vi "build.maps.vi"(8 "error in (no error)":errorcluster, 10 "manager_daemon.lvclass":refnum<class "manager_daemon.lvclass">, 11 "paths":T1={"issue map path"=path "D:/Comics/data/key_maps/issues.bin", "char map path"=path "D:/Comics/data/key_maps/chars.bin", "concept map path"=path "D:/Comics/data/key_maps/concepts.bin", "story map path"=path "D:/Comics/data/key_maps/storys.bin", "team map path"=path "D:/Comics/data/key_maps/teams.bin", "volume map path"=path "D:/Comics/data/key_maps/volumes.bin", "volumes path"=path "D:/Comics/data/cv_volumes", "issues path"=path "D:/Comics/data/cv_issues", "folder map path"=path ""}) -> (0 "error out":errorcluster)   [LabVIEW 2024, in "manager_daemon.lvclass"]
uses:
  manager_daemon/manager_daemon.lvclass
  manager_daemon/type_defs/paths--cluster.ctl
  manager_daemon/type_defs/IssueData--clustrer.ctl
  manager_daemon/type_defs/VolumeData--cluster.ctl
  CV_Shared_Library/volume.type--enum.ctl
  manager_daemon/type_defs/sub-map--map.ctl
  manager_daemon/type_defs/SubData--cluster.ctl
  manager_daemon/private/add.sub.to.map.vi
  CV_Shared_Library/open.local.issue.file.vi
  CV_Shared_Library/open.local.volume.file.vi
  CV_Shared_Library/CV_Shared_Library.lvlib
panel:
  out "total volumes":i32
  out "volume progress":i32(slide) scale=0.0..5644.0
  out "total issues":i32
  out "issue progress":i32(slide) scale=0.0..45513.0
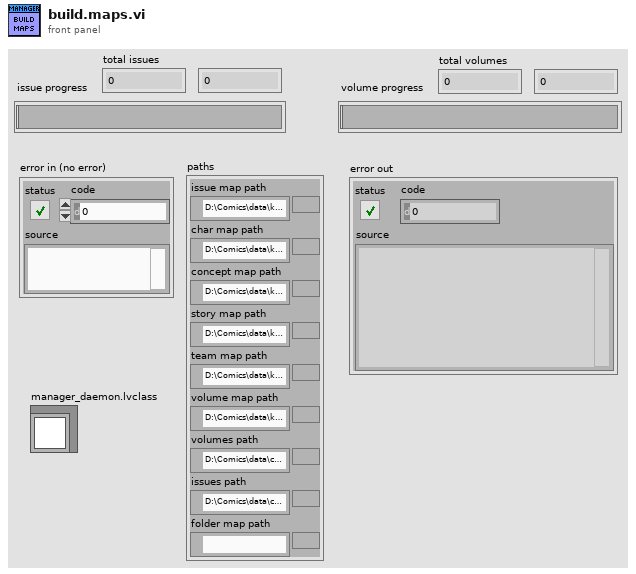
[diagram p1: front panel]
types:
  T1 = typedef "manager_daemon.lvclass/paths--cluster.ctl" = cluster{"issue map path":path, "char map path":path, "concept map path":path, "story map path":path, "team map path":path, "volume map path":path, "volumes path":path, "issues path":path, "folder map path":path}
  T2 = typedef "manager_daemon.lvclass/sub-map--map.ctl" = map{string, T3}
  T3 = typedef "manager_daemon.lvclass/SubData--cluster.ctl" = cluster{"id":i32, "issues":set{i32}}
  T4 = typedef "manager_daemon.lvclass/VolumeData--cluster.ctl" = cluster{"name":string, "sortable_name":string, "aliases":string[], "description":string, "site_detail_url":string, "count_of_issues":i32, "start_year":i32, "publisher_id":i32, "issue_ids":i32[], "date_last_updated":timestamp, "volume":i32, "cv_id":string, "volume type":T5, "source_path":path}
  T5 = typedef "CV_Shared_Library.lvlib/volume.type--enum.ctl" = enum16{"Ongoing", "Limited Series", "Annual", "One Shot", "Reprint/Document", "Star Comics", "Epic Comics"}
  T6 = typedef "manager_daemon.lvclass/IssueData--clustrer.ctl" = cluster{"cover_date":timestamp, "cv_id":string, "name":string, "sortable_name":string, "issue_number":string, "deck":string, "description":string, "id":i32, "store_date":timestamp, "date_last_updated":timestamp, "site_detail_url":string, "cover_url":string, "source_path":path}
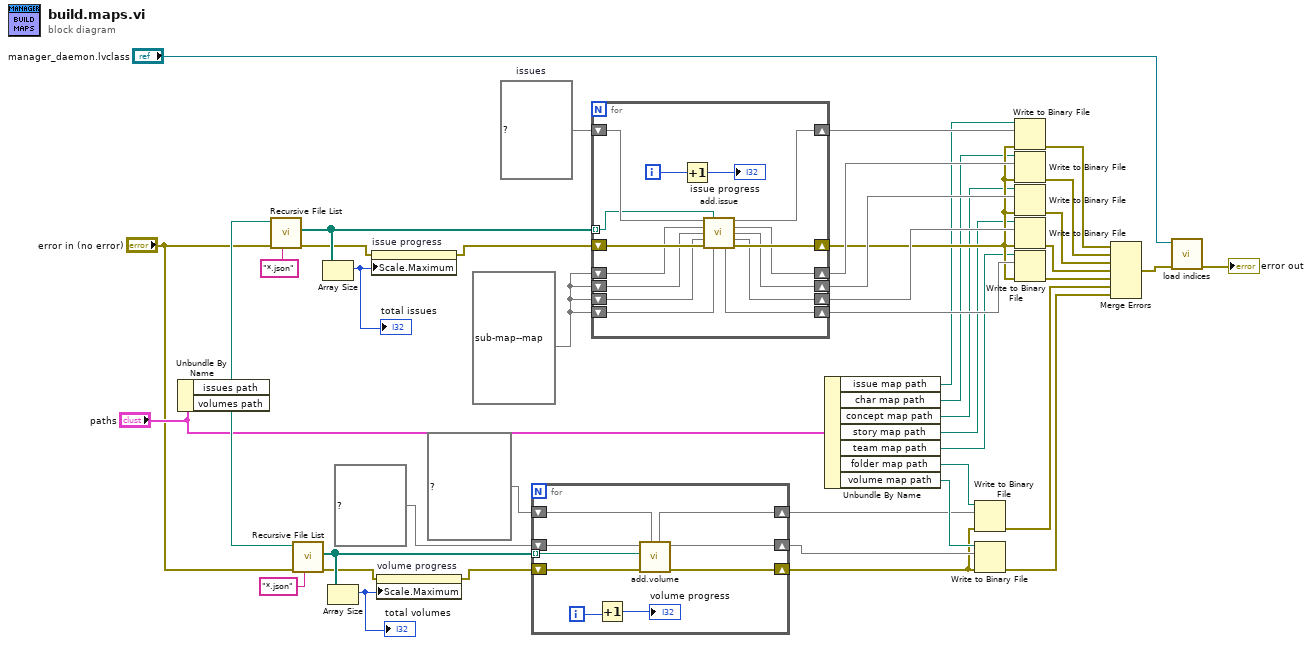
[diagram p0: block diagram]
diagram:
  w11 = T2 {} ("map")
  w43 = map{i32, T6} {}  # issues
  n1 = Unbundle By Name("paths") -> ("issues path"=w22:path, "volumes path"=w19:path)
  n2 = call <vilib>:"Recursive File List.vi"("pattern"="*.json", "error in (no error)"="error in (no error)", "Folder Path"=w22) -> ("error out"=w24:errorcluster, "All Files in Dir"=w42:path[])  [unwired: 4 in, 3 out]
  n3 = call <vilib>:"Recursive File List.vi"("pattern"="*.json", "error in (no error)"="error in (no error)", "Folder Path"=w19) -> ("error out"=w21:errorcluster, "All Files in Dir"=w28:path[])  [unwired: 4 in, 3 out]
  n4 = Array Size(array=w42) -> (size(s)=w41:i32)
  "total issues" <- w41
  n5 = Array Size(array=w28) -> (size(s)=w29:i32)
  "total volumes" <- w29
  n6 = property on="issue progress" class="Slide (strict)"(error in=w24, "Scale.Maximum"=w41) -> (error out=w23:errorcluster)  [unwired: 1 in, 1 out]
  n7 = property on="volume progress" class="Slide (strict)"(error in=w21, "Scale.Maximum"=w29) -> (error out=w20:errorcluster)  [unwired: 1 in, 1 out]
  n8 = for {
    tunnel: w28 -> [w47] mode=indexing
    shift-right: [w49] -> w2
    shift-left: w20 -> [w53]
    shift-right: [w50] -> w25
    shift-left: map{i32, T4} {} ("map") -> [w48]
    shift-right: [w45] -> w5
    shift-left: map{i32, map{string, i32}} {} ("folder map in") -> [w46]
    i -> [w52]
    n9 = Increment(x=w52) -> (x+1=→"volume progress":i32)
    n10 = call "add.volume.vi"("folder map in"=w46, "error in (no error)"=w53, "Path"=w47, "volume map in"=w48) -> ("error out"=w49:errorcluster, "volume map out"=w50:map{i32, T4}, "folder map out"=w45:map{i32, map{string, i32}})  [unwired: 5 in]
  }
  n11 = for {
    tunnel: w42 -> [w59] mode=indexing
    shift-right: [w66] -> w35
    shift-left: w23 -> [w68]
    shift-right: [w54] -> w40
    shift-left: w43 -> [w67]
    shift-right: [w55] -> w39
    shift-left: w11 -> [w65]
    shift-right: [w56] -> w36
    shift-left: w11 -> [w64]
    shift-right: [w57] -> w37
    shift-left: w11 -> [w63]
    shift-right: [w58] -> w38
    shift-left: w11 -> [w62]
    i -> [w61]
    n12 = Increment(x=w61) -> (x+1=→"issue progress":i32)
    n13 = call "add.issue.vi"("issues in"=w67, "Path"=w59, "char map in"=w65, "concept map in"=w64, "story map in"=w63, "error in (no error)"=w68, "team map in"=w62) -> ("issues out"=w54:map{i32, T6}, "char map out"=w55:T2, "concept map out"=w56:T2, "story map out"=w57:T2, "team map out"=w58:T2, "error out"=w66:errorcluster)  [unwired: 3 in]
  }
  n14 = Unbundle By Name("paths") -> ("issue map path"=w13:path, "char map path"=w14:path, "concept map path"=w15:path, "story map path"=w16:path, "team map path"=w17:path, "folder map path"=w4:path, "volume map path"=w6:path)
  n15 = Write to Binary File(file (use dialog)=w4, data=w5, error in=w2) -> (error out=w1:errorcluster)  [unwired: 3 in, 2 out]
  n16 = Write to Binary File(file (use dialog)=w6, data=w25, error in=w2) -> (error out=w3:errorcluster)  [unwired: 3 in, 2 out]
  n17 = Write to Binary File(file (use dialog)=w13, data=w40, error in=w35) -> (error out=w34:errorcluster)  [unwired: 3 in, 2 out]
  n18 = Write to Binary File(file (use dialog)=w14, data=w39, error in=w35) -> (error out=w33:errorcluster)  [unwired: 3 in, 2 out]
  n19 = Write to Binary File(file (use dialog)=w15, data=w36, error in=w35) -> (error out=w27:errorcluster)  [unwired: 3 in, 2 out]
  n20 = Write to Binary File(file (use dialog)=w16, data=w37, error in=w35) -> (error out=w32:errorcluster)  [unwired: 3 in, 2 out]
  n21 = Write to Binary File(file (use dialog)=w17, data=w38, error in=w35) -> (error out=w31:errorcluster)  [unwired: 3 in, 2 out]
  n22 = Merge Errors(w34, w33, w27, w32, w31, w1, w3) -> (w10:errorcluster)
  n23 = call "load indices.vi"("error in (no error)"=w10, "manager_daemon in"="manager_daemon.lvclass") -> ("error out"=→"error out":errorcluster)  [unwired: 8 in, 1 out]
